vi "S8300E_Memory_Test_WIH.vi"() -> ()   [LabVIEW 2011]
panel:
  out "PRELOG2":string
  out "PRELOG1":string
  out "Log":string
  out "MSG List":string[](array[string])
  out "VISA resource name out":refnum<visa-resource-name>
  out "Cmd Line":cluster{string, string, "BIST Version":string}[](array[cluster])
  out "MEMSIZE_SLOT2":string
  out "MEMSIZE_SLOT1":string
  out "BEGIN TIME":u32
  out "進行狀況":string
  # "Error Code:MEMORY\nError Code:UART"
  # "S8300E Memory Check (接UART COM9)"
  # "2015-6-1"
  # "Step1:Memory Type\nStep2:Memory Size\nStep3:Memory Clock\nStep4:Test Memory module ECC status\nStep5: Register value of DIMM1/DIMM2"
  # "Baud-Rate:115200"
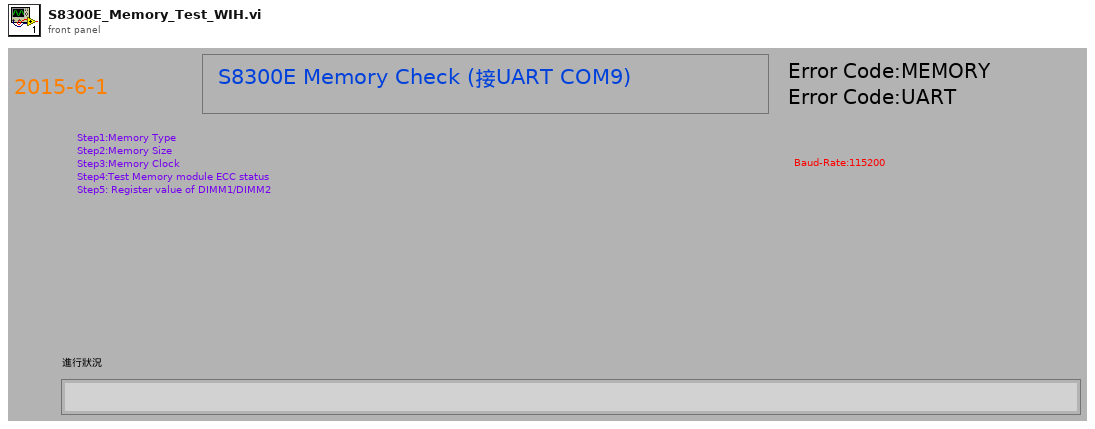
[diagram p1: front panel]
types:
  T1 = cluster{string, string, "MEMSIZE_SLOT2":string}[]
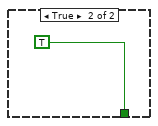
[diagram p5: hidden frame]
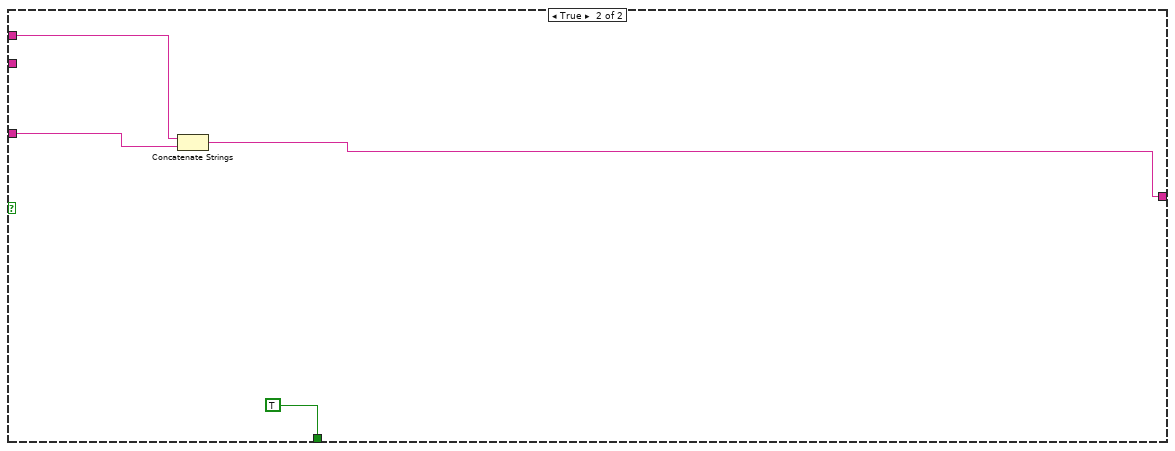
[diagram p8: hidden frame]
diagram:
  n1 = flat-sequence {
    frame #0 {
      n2 = Tick Count (ms)() -> (millisecond timer value=→"BEGIN TIME":u32)
    }
    frame #1 {
      n3 = Request Deallocation(TRUE ("flag")) -> ()
      n4 = property on="進行狀況" class="Str"("Blinking"=TRUE) -> ()  [unwired: 2 in, 2 out]
      "進行狀況" <- "進入測試準備中...." ("進行狀況")
    }
    frame #2 {
      n5 = call "SUB_SearchFile_inFolder.vi"("Search Filename in Folder"="S8300E_sfcs_misc.txt") -> ("File Existing True/Flase"=w5:bool)  [unwired: 1 in]
      n6 = case shown="False" w5 {
        frame False {
          n7 = flat-sequence {
            frame #0 {
              n8 = call "Display Message to User"() -> ()  [unwired: 10 in, 2 out]
            }
            frame #1 {
              n9 = call "SUB_Writelog.vi"("Pass/Fail"="Fail:S8300E_Memory_Test") -> ()  [unwired: 2 in]
            }
            frame #2 {
              n10 = Quit LabVIEW(quit? (T)=TRUE) -> ()
            }
          }
        }
        frame True {
        }
      }
    }
    frame #3 {
      n11 = call "SUB_ReadScript_File.vi"("Script FileName"="S8300E_sfcs_misc.txt" ("Search Filename in Folder")) -> ("text"=w13:string)  [unwired: 1 in, 2 out]
      n12 = call "SUB_FindSpecificString.vi"("Find this String"="UUT_MEMORY_SIZE_SLOT2=", "String data"=w13) -> ("before \"; \" string"=→"MEMSIZE_SLOT2":string, "Found"=w10:bool)  [unwired: 2 in]
      n13 = call "SUB_FindSpecificString.vi"("Find this String"="UUT_MEMORY_SIZE_SLOT1=", "String data"=w13) -> ("before \"; \" string"=→"MEMSIZE_SLOT1":string, "Found"=w11:bool)  [unwired: 2 in]
      n14 = And(x=w11, y=w10) -> (x .and. y?=w9:bool)
      n15 = case shown="False" w9 {
        frame False {
          n16 = flat-sequence {
            frame #0 {
              n17 = call "Display Message to User2"() -> ()  [unwired: 10 in, 2 out]
            }
            frame #1 {
              n18 = call "SUB_Writelog.vi"("Pass/Fail"="Fail:S8300E_Memory_Test") -> ()  [unwired: 2 in]
            }
            frame #2 {
              n19 = Quit LabVIEW(quit? (T)=TRUE) -> ()
            }
          }
        }
        frame True {
        }
      }
    }
    frame #4 {
      w48 = "1600 MHz"  # 1600 MHz
      w51 = "1600 MHz"  # 1600 MHz
      n20 = local read "MEMSIZE_SLOT2"() -> (w35:string)
      n21 = local read "MEMSIZE_SLOT1"() -> (w36:string)
      n22 = Bundle("./mem.sh -t 1", "PASSED=", "DDR3") -> (w47:cluster{string, string, string})  [unwired: 1 in]
      n23 = Bundle("./mem.sh -t 2", "PASSED=", "DDR3") -> (w46:cluster{string, string, string})  [unwired: 1 in]
      n24 = Bundle("./mem.sh -s 1", "PASSED=", "MEMSIZE_SLOT1"=w36) -> (w45:cluster{string, string, "MEMSIZE_SLOT1":string})  [unwired: 1 in]
      n25 = Bundle("./mem.sh -c  1", "PASSED=", w51) -> (w43:cluster{string, string, string})  [unwired: 1 in]
      n26 = Bundle("i2cget -y 0 0x52 0x03", "0x08", "") -> (w22:cluster{string, string, string})  [unwired: 1 in]
      n27 = Bundle("./mem.sh -s  2", "PASSED=", "MEMSIZE_SLOT2"=w35) -> (w44:cluster{string, string, "MEMSIZE_SLOT2":string})  [unwired: 1 in]
      n28 = Bundle("./mem.sh -c  2", "PASSED=", w48) -> (w42:cluster{string, string, string})  [unwired: 1 in]
      n29 = Bundle("i2cget -y 0 0x50 0x03 ", "0x08", "") -> (w23:cluster{string, string, string})  [unwired: 1 in]
      n30 = Bundle("./mem.sh -e", "PASSED=", "") -> (w31:cluster{string, string, string})  [unwired: 1 in]
      n31 = Build Array("處理Memory Type Slot 1", "處理Memory Type Slot 2", "處理Memory Size Slot 1", "處理Memory Size  Slot 2", "處理Memory Clock   Slot 1", "處理Memory Clock  Slot 2", "處理Test Memory module ECC status", "0x08;檢查 Register Value of DMM1...", "0x08;檢查  Register Value of DMM2...") -> (→"MSG List":string[])
      n32 = Build Array(w47, w46, w45, w44, w43, w42, w31, w23, w22) -> (→"Cmd Line":T1)
    }
    frame #5 {
      n33 = call "SUB_COM1_CLOSE.vi"("VISA resource name"=refnum<visa-resource-name> "COM9") -> ()  [unwired: 3 in]
    }
    frame #6 {
      n34 = call "SUB_COM9_INIT.vi"("baud rate"=u32 115200) -> ("VISA resource name out"=w71:refnum<visa-resource-name>)  [unwired: 1 in, 1 out]
      "VISA resource name out" <- w71
      n35 = call "SUB_COM1Wrt.vi"("VISA resource name"=w71, "write buffer"="\r") -> ("duplicate VISA resource name"=w68:refnum<visa-resource-name>)  [unwired: 1 in, 1 out]
      n36 = call "SUB_ContinueCom1Read.vi"("Numeric"=1200, "duplicate VISA resource name 2"=w68) -> ()  [unwired: 1 in, 3 out]
    }
    frame #7 {
      n37 = while {
        stop <- w83 stop-if-true
        w81 = "\r"
        n38 = local read "VISA resource name out"() -> (w74:refnum<visa-resource-name>)
        n39 = Concatenate Strings(w81, w81, w81) -> (w80:string)
        n40 = call "SUB_ContinueCom1Read.vi"("Numeric"=1200, "duplicate VISA resource name 2"=w74) -> ("duplicate VISA resource name"=w73:refnum<visa-resource-name>)  [unwired: 1 in, 2 out]
        n41 = Tick Count (ms)() -> (millisecond timer value=w82:u32)
        n42 = call "SUB_WR_COM1_CbyCFindString_timeout.vi"("Begin time"=w82, "Find this String"="S8300E", "Timeout Seccond"=3.0, "cmd string"=w80, "duplicate VISA resource name 2"=w73) -> ("Output String"=w77:string, "Found String"=w76:bool)  [unwired: 2 out]
        n43 = case shown="False" w76 {
          tunnel: w77 -> [w88 _]
          tunnel: [w84 TRUE] -> w83
          frame False {
            n44 = call "SUB_YESNO.vi"("Debug View"=w88, "Status"="UART無正確反應!需有S8300E字串") -> ("yes/no"=w87:enum32{"No Selection", "Yes", "No", "None"})  [unwired: 1 in]
            n45 = Equal?(x=w87, y=enum32{"No Selection", "Yes", "No", "None"}."No") -> (x = y?=w85:bool)
            n46 = case shown="True" w85 {
              tunnel: [_ w90] -> w84
              frame False {
              }
              frame True {
                n47 = flat-sequence {
                  tunnel: [w94] -> w90
                  frame #0 {
                    n48 = call "SUB_Writelog.vi"("Pass/Fail"="Fail:S8300E_Memory_Test") -> ()  [unwired: 2 in]
                  }
                  frame #1 {
                    n49 = call "SUB_SFCS_SendResult.vi"("ErrorCode"="UART", "PASS_Fail (1/0)"=i8 0) -> ()  [unwired: 1 out]
                  }
                  frame #2 {
                    w94 = TRUE ("quit? (T)")
                    n50 = Quit LabVIEW(quit? (T)=w94) -> ()
                  }
                }
              }
            }
          }
          frame True {
          }
        }
      }
    }
    frame #8 {
      n51 = local read "Cmd Line"() -> (w99:cluster{string, string, "BIST Version":string}[])
      n52 = Array Size(array=w99) -> (size(s)=w98:i32)
      n53 = for {
        N: w98 -> [_]
        shift-right: [w101] -> w96
        shift-left: "" -> [w100]
        i -> [w104]
        n54 = while {
          tunnel: w104 -> [w133]
          shift-right: [w110] -> w102
          shift-left: "" -> [w109]
          stop <- w129 stop-if-true
          n55 = local read "VISA resource name out"() -> (w112:refnum<visa-resource-name>)
          n56 = local read "Cmd Line"() -> (w132:cluster{string, string, "BIST Version":string}[])
          n57 = call "SUB_ContinueCom1Read.vi"("Numeric"=1200, "duplicate VISA resource name 2"=w112) -> ("duplicate VISA resource name"=w111:refnum<visa-resource-name>)  [unwired: 1 in, 2 out]
          n58 = Index Array(array=w132, index=w133) -> (element=w131:cluster{string, string, "BIST Version":string})
          n59 = Tick Count (ms)() -> (millisecond timer value=w122:u32)
          n60 = Unbundle(w131) -> (w125:string, w123:string, "BIST Version"=w119:string)
          n61 = Concatenate Strings(w125, "\r") -> (w108:string)
          n62 = call "SUB_COM1Wrt.vi"("VISA resource name"=w111, "write buffer"=w108) -> ("duplicate VISA resource name"=w124:refnum<visa-resource-name>)  [unwired: 1 in, 1 out]
          n63 = call "SUB_READ_COM1_FindString_timeout.vi"("Find this String"=w123, "Timeout Seccond"=2.0, "Begin time"=w122, "duplicate VISA resource name 2"=w124) -> ("Output String"=w120:string)  [unwired: 1 in, 2 out]
          n64 = To Upper Case(1:w119) -> (0:w118:string)
          n65 = call "SUB_FindSpecificString.vi"("Find this String"=w123, "String data"=w120) -> ("before \"; \" string"=w130:string, "Found"=w127:bool)  [unwired: 2 in]
          n66 = Equal?(x=w118, y="") -> (x = y?=w116:bool)
          n67 = Equal?(x=w130, y=w118) -> (x = y?=w114:bool)
          n68 = case shown="True" w116 {
            tunnel: [w134 TRUE] -> w115
            tunnel: w114 -> [w134 _]
            frame False {
            }
            frame True {
            }
          }
          n69 = And(x=w127, y=w115) -> (x .and. y?=w128:bool)
          n70 = case shown="False" w128 {
            tunnel: [_ TRUE] -> w129
            tunnel: w120 -> [w138 w161]
            tunnel: w118 -> [w143 _]
            tunnel: w108 -> [_ w160]
            tunnel: [w136 w159] -> w107
            frame False {
              n71 = local read "進行狀況"() -> (w141:string)
              n72 = Concatenate Strings("版本與定義不符合!系統需回傳  " ("string"), w143, "\r", w141) -> (w140:string)
              n73 = call "SUB_YESNO.vi"("Debug View"=w138, "Status"=w140) -> ("yes/no"=w147:enum32{"No Selection", "Yes", "No", "None"})  [unwired: 1 in]
              n74 = Equal?(x=w147, y=enum32{"No Selection", "Yes", "No", "None"}."No") -> (x = y?=w144:bool)
              n75 = Concatenate Strings(w140, "\r", w138) -> (w137:string)
              n76 = case shown="True" w144 {
                tunnel: w137 -> [w148 w149]
                tunnel: [w148 _] -> w136
                frame False {
                }
                frame True {
                  n77 = flat-sequence {
                    tunnel: w149 -> [w150]
                    tunnel: [w158] -> _
                    frame #0 {
                      w152 = "\r"
                      n78 = local read "PRELOG2"() -> (w154:string)
                      n79 = local read "PRELOG1"() -> (w153:string)
                      n80 = Concatenate Strings("Fail:S8300E_Memory_Test" ("Pass/Fail"), w152, w154, w152, w153, w152, w150) -> (w151:string)
                      n81 = call "SUB_Writelog.vi"("Pass/Fail"=w151) -> ()  [unwired: 2 in]
                    }
                    frame #1 {
                      n82 = call "SUB_SFCS_SendResult.vi"("ErrorCode"="MEMORY", "PASS_Fail (1/0)"=i8 0) -> ()  [unwired: 1 out]
                    }
                    frame #2 {
                      w158 = TRUE ("quit? (T)")
                      n83 = Quit LabVIEW(quit? (T)=w158) -> ()
                    }
                  }
                }
              }
            }
            frame True {
              n84 = Concatenate Strings(w160, w161) -> (w159:string)
            }
          }
          n85 = Concatenate Strings(w109, w107) -> (w110:string)
          "PRELOG1" <- w110
        }
        n86 = local read "MSG List"() -> (w106:string[])
        n87 = Index Array(array=w106, index=w104) -> (element=w105:string)
        n88 = local write "進行狀況"(w105) -> ()
        n89 = Concatenate Strings(w100, w102) -> (w101:string)
        "PRELOG2" <- w101
      }
      "Log" <- w96
    }
    frame #9 {
      n90 = call "SUB_COM1_CLOSE.vi"("VISA resource name"=refnum<visa-resource-name> "COM9") -> ()  [unwired: 3 in]
    }
    frame #10 {
      w166 = "***Not Good ***" ("replace string (\"\")")
      n91 = local read "BEGIN TIME"() -> (w175:u32)
      n92 = Tick Count (ms)() -> (millisecond timer value=w174:u32)
      n93 = call "SUB_CAL_TESTTIME.vi"("Test Item name"="S8300E_Memory_Test", "Stop tick time"=w174, "Start tick time"=w175) -> ("Test Time output"=w170:string)  [unwired: 2 in]
      n94 = local read "Log"() -> (w171:string)
      n95 = Concatenate Strings("Pass:S8300E_Memory_Test", "\n", w171, w170) -> (w165:string)
      n96 = call "SUB_SEARCH_REPLACE_STR.vi"("replace string (\"\")"=w166, "search string"="FAILED", "input string"=w165) -> ("result string"=w168:string)  [unwired: 2 in]
      n97 = call "SUB_SEARCH_REPLACE_STR.vi"("replace string (\"\")"=w166, "search string"="FAIL", "input string"=w168) -> ("result string"=w164:string)  [unwired: 2 in]
      n98 = call "SUB_Writelog.vi"("Pass/Fail"=w164) -> ()  [unwired: 2 in]
    }
    frame #11 {
      n99 = Request Deallocation(TRUE ("flag")) -> ()
    }
    frame #12 {
      n100 = Quit LabVIEW(quit? (T)=TRUE ("stop? (T)")) -> ()
    }
  }
